vi "TailInsertionBenchmark.vi"() -> ()   [LabVIEW 2009]
uses:
  ImpSelectionEnum.ctl
  source/Lists/ListImp/ListImp.lvclass
  source/Lists.Implementations/BufferedArray/BufferedArray.lvclass
  source/Lists.Interfaces/StringList/StringList.lvclass
panel:
  in  "Number of Elements":i32
  in  "Implementation":T1
  out "Buffered Array List Imp":u32
  out "Default List Imp":u32
  out "error out":errorcluster
  # "Tail Insertion"
  # "100,000 to 500,000 elements is sufficient to see the difference in time for each of the implementations."
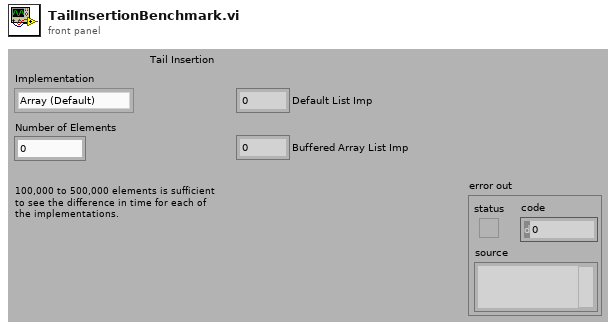
[diagram p1: front panel]
types:
  T1 = typedef "ImpSelectionEnum.ctl" = enum16{"Array (Default)", "Buffered Array"}
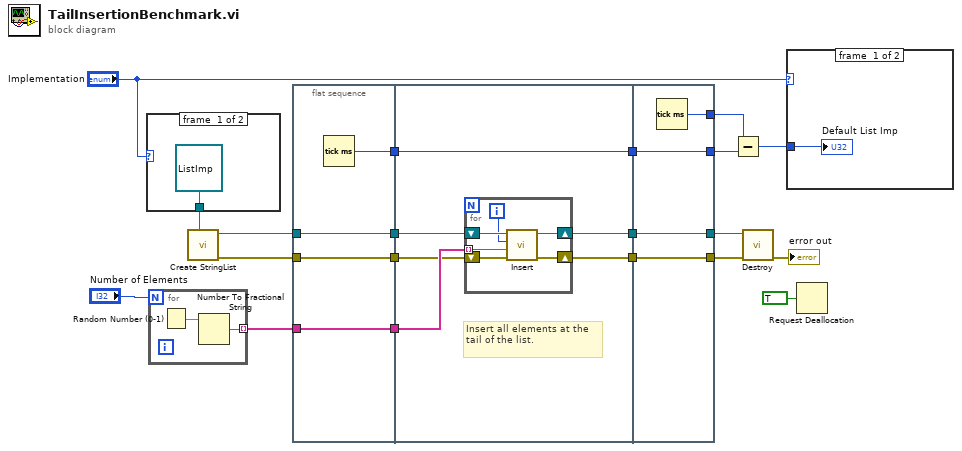
[diagram p0: block diagram]
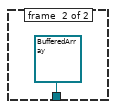
[diagram p2: hidden frame]
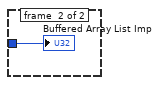
[diagram p3: hidden frame]
diagram:
  n1 = case shown="\"Array (Default)\", Default" "Implementation" {
    tunnel: [refnum<class "ListImp.lvclass"> refnum ("LapDog.Collections.v0.Lists.lvlib:ListImp.lvclass") refnum<class "BufferedArray.lvclass"> refnum ("LapDog.Collections.v0.Lists.Implementations.lvlib:BufferedArray.lvclass")] -> w16
    frame #0 {
    }
    frame #1 {
    }
  }
  n2 = for {
    N: "Number of Elements" -> [_]
    tunnel: [w23] -> w19 mode=indexing
    n3 = Random Number (0-1)() -> (number: 0 to 1=w24:dbl)
    n4 = Number To Fractional String(number=w24) -> (F-format string=w23:string)  [unwired: 3 in]
  }
  n5 = call "Create StringList.vi"("List Implementation (Array)"=w16) -> ("error out"=w12:errorcluster, "StringList out"=w14:refnum<class "StringList.lvclass">)  [unwired: 9 in]
  n6 = flat-sequence {
    tunnel: w19 -> [w28]
    tunnel: [w28] -> w18
    tunnel: [w27] -> w17
    tunnel: [w26] -> w15
    tunnel: w14 -> [w26]
    tunnel: [w25] -> w13
    tunnel: w12 -> [w25]
    tunnel: w18 -> [w34]
    tunnel: w17 -> [w29]
    tunnel: w15 -> [w33]
    tunnel: w13 -> [w32]
    tunnel: [w31] -> w11
    tunnel: [w30] -> w10
    tunnel: [w29] -> w9
    tunnel: [w43] -> w6
    tunnel: [w44] -> w5
    tunnel: w11 -> [w44]
    tunnel: w10 -> [w43]
    tunnel: w9 -> [w41]
    tunnel: [w42] -> w8
    tunnel: [w41] -> w7
    frame #0 {
      n7 = Tick Count (ms)() -> (millisecond timer value=w27:u32)
    }
    frame #1 {
      # "Insert all elements at the tail of the list."
      n8 = for {
        shift-right: [w39] -> w31
        shift-left: w33 -> [w40]
        tunnel: w34 -> [w38] mode=indexing
        shift-right: [w35] -> w30
        shift-left: w32 -> [w36]
        i -> [w37]
        n9 = call-dynamic "Insert.vi"("error in (no error)"=w36, "String"=w38, "Index"=w37, "StringList in"=w40) -> ("error out"=w35:errorcluster, "StringList out"=w39:refnum<class "StringList.lvclass">)  [unwired: 6 in]
      }
    }
    frame #2 {
      n10 = Tick Count (ms)() -> (millisecond timer value=w42:u32)
    }
  }
  n11 = Subtract(x=w8, y=w7) -> (x-y=w3:u32)
  n12 = call-dynamic "Destroy.vi"("error in (no error)"=w6, "StringList in"=w5) -> ("error out"=→"error out":errorcluster)  [unwired: 9 in]
  n13 = case shown="\"Array (Default)\", Default" "Implementation" {
    tunnel: w3 -> [w45 w46]
    frame #0 {
      "Default List Imp" <- w45
    }
    frame #1 {
      "Buffered Array List Imp" <- w46
    }
  }
  n14 = Request Deallocation(TRUE ("flag")) -> ()
